vi "Database Check.vi"(6 "Menu ref":refnum<k9>, 8 "error in (no error)":errorcluster, 9 "Database status ref":refnum<vi>, 10 "Array ref in":refnum<vi>[](array[refnum]), 11 "Database not available for at least one?":bool) -> (0 "error out":errorcluster)   [LabVIEW 2014]
doc: "<B>Copyright</B>: (c) MHWirth 2015. All rights are reserved.\n\nThis subVI controls the \"enable\" state of Create Database button, and updates the Database Status."
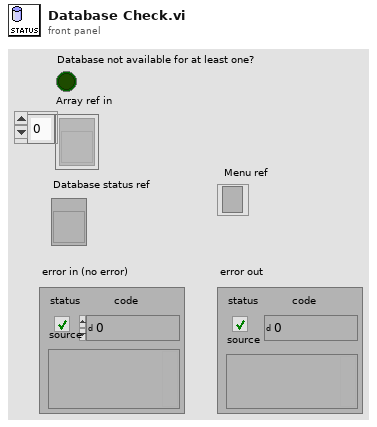
[diagram p1: front panel]
types:
  T1 = enum8{"Enabled", "Disabled", "Disabled and Grayed Out"}
  T2 = enum8{"Enabled", "Disabled", "Disabled and Grayed Out"}[]
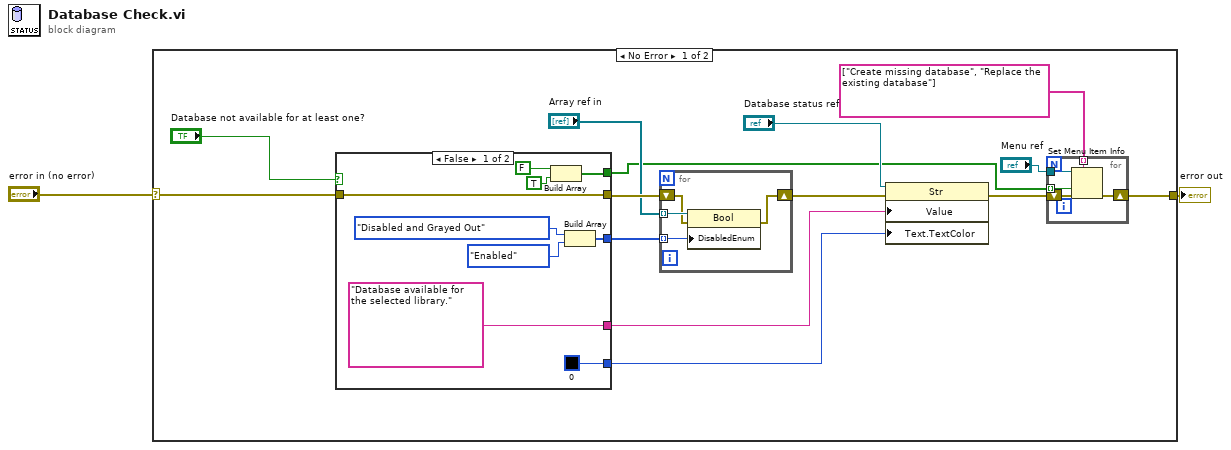
[diagram p0: block diagram]
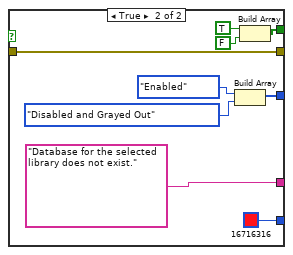
[diagram p2: hidden frame]
diagram:
  n1 = case shown="No Error" "error in (no error)" {
    selector: "error in (no error)" -> [w16 w44]
    tunnel: [w6 w44] -> w1
    frame No Error {
      n2 = case shown="False" "Database not available for at least one?" {
        tunnel: ["Database available for the selected library." "Database for the selected library does not exist."] -> w9
        tunnel: w16 -> [w30 w39]
        tunnel: [w31 w40] -> w14
        tunnel: [w30 w39] -> w13
        tunnel: [u32 0 u32 16716316] -> w8
        tunnel: [w28 w36] -> w4
        frame False {
          n3 = Build Array(FALSE, TRUE ("element")) -> (w28:bool[])
          n4 = Build Array(T1."Disabled and Grayed Out" ("Disabled"), T1."Enabled" ("Disabled")) -> (w31:T2)
        }
        frame True {
          n5 = Build Array(T1."Enabled" ("Disabled"), T1."Disabled and Grayed Out" ("Disabled")) -> (w40:T2)
          n6 = Build Array(TRUE, FALSE ("element")) -> (w36:bool[])
        }
      }
      n7 = for {
        tunnel: "Array ref in" -> [w25] mode=indexing
        tunnel: w14 -> [w24] mode=indexing
        shift-right: [w22] -> w10
        shift-left: w13 -> [w23]
        n8 = property class="Bool"(reference=w25, error in=w23, "DisabledEnum"=w24) -> (error out=w22:errorcluster)  [unwired: 1 out]
      }
      n9 = property on="Property Node" class="Str"(reference="Database status ref", error in=w10, "Value"=w9, "Text.TextColor"=w8) -> (error out=w7:errorcluster)  [unwired: 1 out]
      n10 = for {
        tunnel: "Menu ref" -> [w19]
        tunnel: string[] ["Create missing database", "Replace the existing database"] -> [w18] mode=indexing
        tunnel: w4 -> [w17] mode=indexing
        shift-right: [w20] -> w6
        shift-left: w7 -> [w21]
        n11 = Set Menu Item Info(7:w18, 8:w21, 9:w17, 11:w19) -> (0:w20:errorcluster)  [unwired: 3 in, 1 out]
      }
    }
    frame Error {
    }
  }
  "error out" <- w1
